vi "Restore Panel (by name).vi"(8 "Error In":errorcluster, 9 "Name":string, 10 "VI reference":refnum<vi>, 11 "Path (dialog)":path=path "C:/ProgramData/EPL/CFTS Defaults.ini") -> (0 "error out":errorcluster)   [LabVIEW 2020]
doc: "Attempt to restore panel controls from a file.\n\nFreeware from Moore Good Ideas, www.mooregoodideas.com. Do not remove this line.\ndavid@mooregoodideas.com"
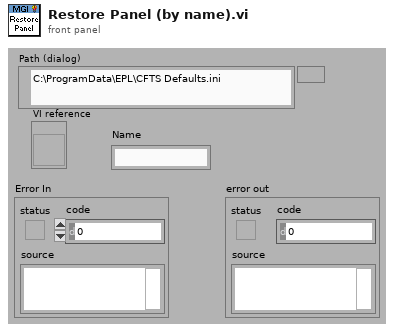
[diagram p1: front panel]
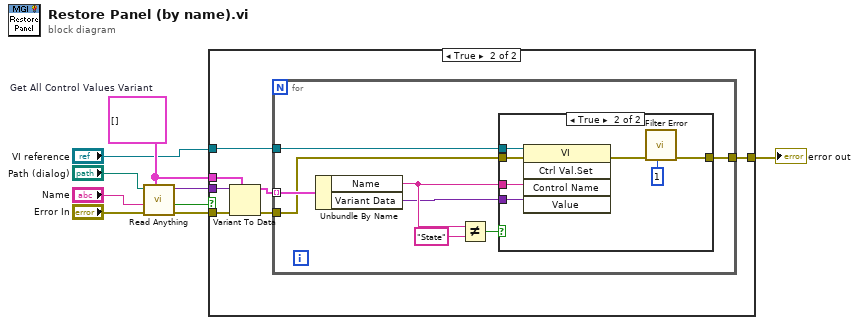
[diagram p0: block diagram]
diagram:
  w9 = cluster{"Name":string, "Variant Data":variant}[] []  # Get All Control Values Variant
  n1 = call "Read Anything.vi"("Type of Anything"=w9, "Error In"="Error In", "Section Name (Name of \"Type of Anything\")"="Name", "Path (dialog)"="Path (dialog)") -> ("Error Out"=w7:errorcluster, "Found?"=w5:bool, "Anything"=w8:variant)  [unwired: 5 out]
  n2 = case shown="True" w5 {
    tunnel: w9 -> [_ w15]
    tunnel: w8 -> [_ w14]
    tunnel: w7 -> [w10 w13]
    tunnel: "VI reference" -> [_ w12]
    tunnel: [w10 w11] -> w6
    frame False {
    }
    frame True {
      n3 = Variant To Data(error in=w13, type=w15, Variant=w14) -> (data=w16:cluster{"Name":string, "Variant Data":variant}[], error out=w17:errorcluster)
      n4 = for {
        tunnel: w16 -> [w25] mode=indexing
        tunnel: w12 -> [w24]
        tunnel: w17 -> [w23]
        tunnel: [w19] -> w11
        n5 = Unbundle By Name(w25) -> ("Name"=w21:string, "Variant Data"=w18:variant)
        n6 = Not Equal?(x=w21, y="State") -> (x != y?=w20:bool)
        n7 = case shown="True" w20 {
          tunnel: w18 -> [_ w33]
          tunnel: w24 -> [_ w32]
          tunnel: w23 -> [w26 w31]
          tunnel: w21 -> [_ w30]
          tunnel: [w26 w28] -> w19
          frame False {
          }
          frame True {
            n8 = invoke class="VI" method="Ctrl Val.Set"(reference=w32, error in=w31, "Control Name"=w30, "Value"=w33) -> (error out=w29:errorcluster)  [unwired: 1 in, 4 out]
            n9 = call "Filter Error.vi"("error in (no error)"=w29, "code to ignore"=1) -> ("error out"=w28:errorcluster)  [unwired: 9 in]
          }
        }
      }
    }
  }
  "error out" <- w6
